vi "Color Pattern Matching.vi"() -> ()   [LabVIEW 2014]
doc: "This example shows how to use the color pattern matching tools in NI Vision.\n\nYou use color pattern matching to locate known reference or fiducial patterns in an image quickly. Pattern matching is the key to many applications. Color pattern matching can provide your application with information about the presence or absence, number, and location of the model within an image.\n\nYou use color pattern matching in the following three general applications areas:\n\n* Alignment -- Determine the position and orientation of a known object by locating features. You use the features as points of reference on the object.\n\n* Gauging -- Measure lengths, diameters, angles, and other critical dimensions. If the measurements fall outside of set tolerance levels, the component is rejected. You sometimes use gauging in-line with the manufacturing process and off-line. If you make the measurements off-line, a sample of components is used to determine the quality of a lot or batch of manufactured components.\n\n* Inspection -- Detect simple flaws, such as missing parts or unreadable printing."
uses:
  <vilib>/vision/NI_Vision_Development_Module.lvlib
panel:
  out "Number of Matches":i32
  out "Results":T1(array[cluster]) {"Position"."Y" format="%.2f"; "Position"."X" format="%.2f"}
  in  "Max # of Matches":i32=5
  in  "Minimum Score":sgl=700.0
  out "Template":T2(plugin-control)
  in  "Stop":bool
  out "Image":T2(plugin-control)
  # "Overview: Demonstrates how to perform Color Pattern Matching using two steps that include learning the color pattern template defined by a Region of Interest (ROI) and then matching the learned template in the image.\nRequirements: Vision Development Software.\nInstructions:\n1. Run the VI.\n2. Draw a ROI in the image to define the template. The learned template is displayed in the Template display and the match results are overlaid on the Image display."
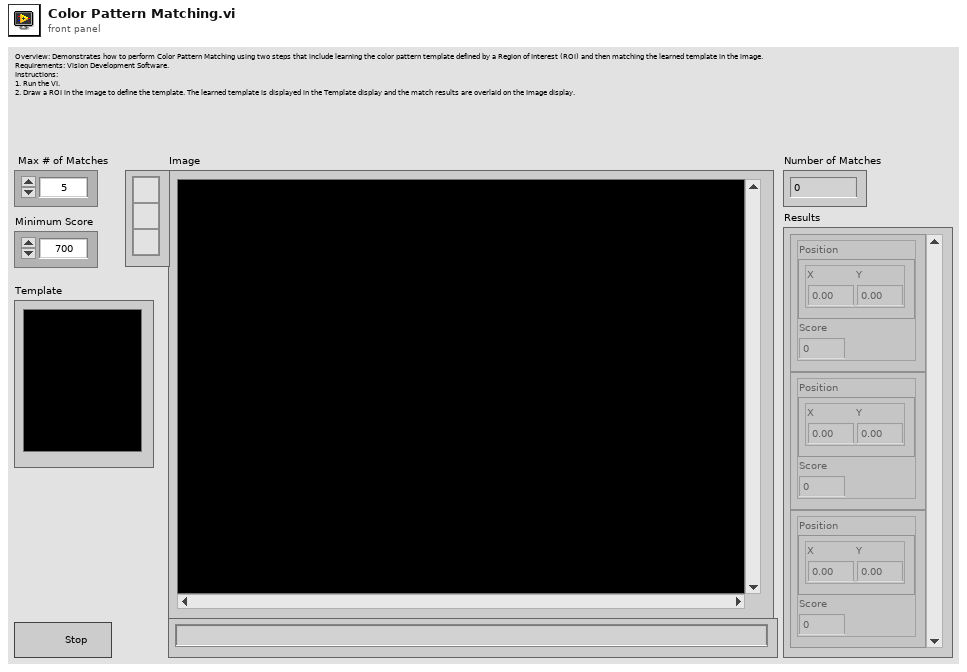
[diagram p1: front panel]
types:
  T1 = cluster{"Position":cluster{"X":dbl, "Y":dbl}, "Score":dbl}[]
  T2 = typedef "IMAQ Image.ctl" = refnum<image>
  T3 = typedef "Image Type" = u32
  T4 = typedef "IMAQ Rectangle" = cluster{"Left":i32, "Top":i32, "Right":i32, "Bottom":i32, "Rotation":dbl}
  T5 = typedef "ROI Descriptor" = cluster{"Global Rectangle":i32[], "Contours":cluster{"ID":enum32{"External", "Internal"}, "Type":u32, "Coordinates":i32[]}[]}
  T6 = cluster{"Max # of Matches":i32, "Minimum Score":sgl}
  T7 = cluster{"Position":cluster{"x":sgl, "y":sgl}, "Angle":sgl, "Scale":sgl, "Score":sgl, "Bounding Box":cluster{"x":sgl, "y":sgl}[]}[]
  T8 = cluster{"Position":cluster{"x":sgl, "y":sgl}, "Score":sgl}
  T9 = cluster{i32[], cluster{"Contour Type":u32, "ROI Type":u32, i32[]}[]}
  T10 = cluster{"Global Rectangle":i32[], "Contours":cluster{"Contour Type":u32, "ROI Type":u32, "Points":i32[]}[]}
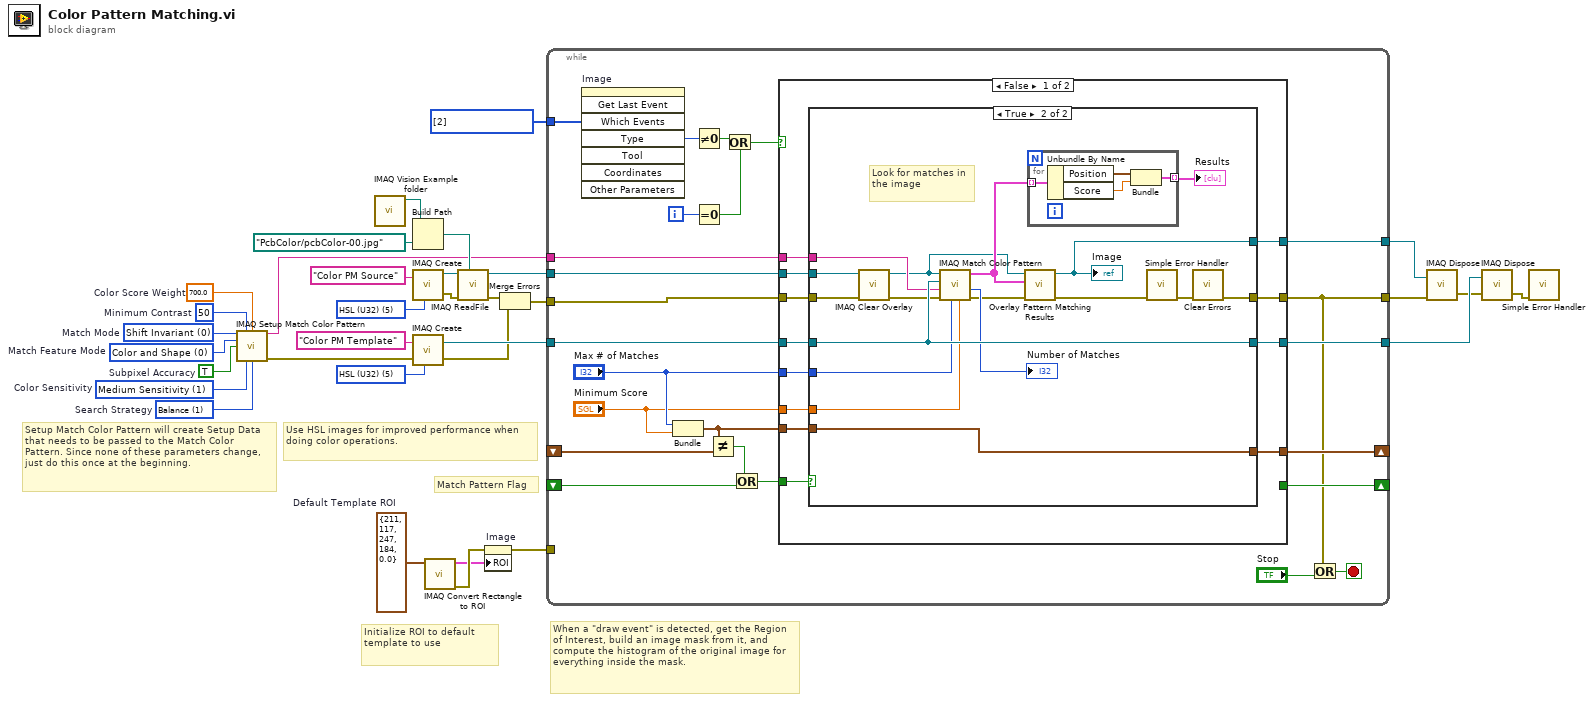
[diagram p0: block diagram]
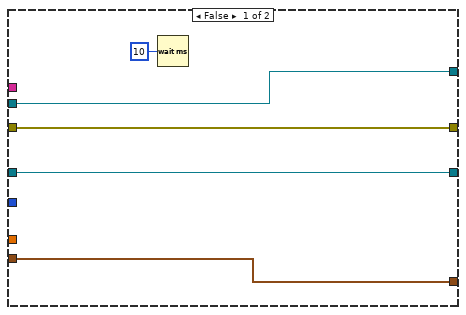
[diagram p2: hidden frame]
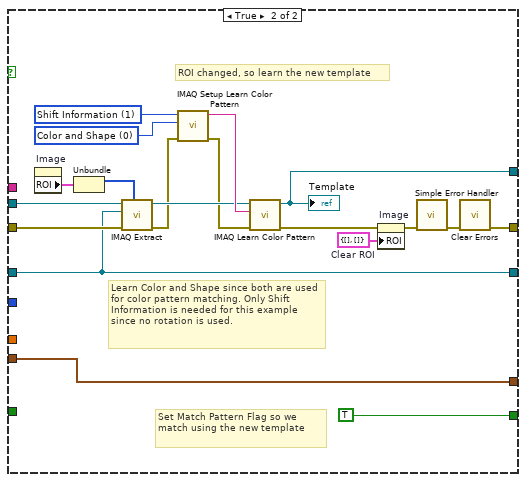
[diagram p3: hidden frame]
diagram:
  w1 = TRUE  # Subpixel Accuracy
  w9 = u32 0 items=["Color and Shape", "Color", "Shape"]  # Match Feature Mode
  w8 = u32 1 items=["Conservative", "Balance", "Aggressive", "Very Aggressive"]  # Search Strategy
  w7 = 50  # Minimum Contrast
  w6 = sgl 700.0  # Color Score Weight
  w5 = u32 1 items=["Low Sensitivity", "Medium Sensitivity", "High Sensitivity"]  # Color Sensitivity
  w4 = u32 0 items=["Shift Invariant", "Rotation Invariant"]  # Match Mode
  w21 = T3 5 items=["Grayscale (U8)", "Grayscale (I16)", "Grayscale (SGL)", "Complex (CSG)", "RGB (U32)", "HSL (U32)", "RGB (U64)", "Grayscale (U16)"] ("Image Type")
  w22 = T3 5 items=["Grayscale (U8)", "Grayscale (I16)", "Grayscale (SGL)", "Complex (CSG)", "RGB (U32)", "HSL (U32)", "RGB (U64)", "Grayscale (U16)"] ("Image Type")
  w27 = i32[] [2] items=["No Event"=0, "Click Event"=1, "Draw Event"=2, "Size Event"=4, "Scroll Event"=5, "Double Click Event"=8] ("Which Events")
  w29 = T4 {"Left"=211, "Top"=117, "Right"=247, "Bottom"=184, "Rotation"=0.0}  # Default Template ROI
  # "Setup Match Color Pattern will create Setup Data that needs to be passed to the Match Color Pattern. Since none of these parameters change, just do this once at the beginning."
  # "Initialize ROI to default template to use"
  # "When a \"draw event\" is detected, get the Region of Interest, build an image mask from it, and compute the histogram of the original image for everything inside the mask."
  # "Match Pattern Flag"
  # "Use HSL images for improved performance when doing color operations."
  n1 = call "IMAQ Setup Match Color Pattern"("Match Mode"=w4, "Minimum Contrast"=w7, "Color Score Weight"=w6, "Match Feature Mode"=w9, "Subpixel Accuracy"=w1, "Color Sensitivity"=w5, "Search Strategy"=w8) -> ("Match Color Pattern Setup Data"=w2:string, "error out"=w3:errorcluster)  [unwired: 7 in]
  n2 = call "IMAQ Vision Example folder.vi"() -> ("Example Image Path"=w32:path)  [unwired: 11 in]
  n3 = Build Path(base path=w32, name or relative path=path "PcbColor/pcbColor-00.jpg") -> (appended path=w28:path)
  n4 = call "IMAQ Create"("Image Name"="Color PM Source", "Image Type"=w22) -> ("New Image"=w13:T2, "error out"=w18:errorcluster)  [unwired: 3 in]
  n5 = call "IMAQ Create"("Image Name"="Color PM Template", "Image Type"=w21, "error in (no error)"=w3) -> ("New Image"=w26:T2, "error out"=w15:errorcluster)  [unwired: 2 in]
  n6 = call "IMAQ Convert Rectangle to ROI"("Rectangle"=w29) -> ("error out"=w17:errorcluster, "ROI Descriptor"=w11:T5)  [unwired: 8 in]
  n7 = call "IMAQ ReadFile"("File Path"=w28, "error in (no error)"=w18, "Image"=w13) -> ("error out"=w16:errorcluster, "Image Out"=w12:T2)  [unwired: 4 in, 3 out]
  n8 = property on="Image" class="ImageControl"(error in=w17, "ROI"=w11) -> (error out=w10:errorcluster)  [unwired: 1 in, 1 out]
  n9 = Merge Errors(w16, w15) -> (w14:errorcluster)
  n10 = while {
    tunnel: w12 -> [w47]
    tunnel: w27 -> [w57]
    tunnel: w26 -> [w46]
    tunnel: w14 -> [w51]
    shift-right: [w45] -> _
    shift-left: _ -> [w38]
    shift-right: [w50] -> _
    shift-left: _ -> [w49]
    tunnel: [w43] -> w25
    tunnel: [w44] -> w24
    tunnel: [w36] -> w23
    tunnel: w10 -> [_]
    tunnel: w2 -> [w40]
    i -> [w54]
    stop <- w34 stop-if-true
    n11 = invoke on="Image" class="ImageControl" method="Get Last Event"("Which Events"=w57) -> ("Type"=w56:i32)  [unwired: 7 in, 7 out]
    n12 = Bundle("Max # of Matches"="Max # of Matches", "Minimum Score"="Minimum Score") -> (w39:T6)  [unwired: 1 in]
    n13 = Not Equal To 0?(x=w56) -> (x != 0?=w55:bool)
    n14 = Equal To 0?(x=w54) -> (x = 0?=w53:bool)
    n15 = Not Equal?(x=w39, y=w38) -> (x != y?=w37:bool)
    n16 = Or(x=w55, y=w53) -> (x .or. y?=w52:bool)
    n17 = Or(x=w37, y=w49) -> (x .or. y?=w48:bool)
    n18 = case shown="False" w52 {
      tunnel: w47 -> [w67 w105]
      tunnel: w51 -> [w66 w104]
      tunnel: w46 -> [w65 w97]
      tunnel: [_ TRUE] -> w50
      tunnel: w48 -> [w69 _]
      tunnel: w39 -> [w68 w96]
      tunnel: [w64 w100] -> w36
      tunnel: [w63 w96] -> w45
      tunnel: [w62 w97] -> w44
      tunnel: [w61 w98] -> w43
      tunnel: "Max # of Matches" -> [w60 _]
      tunnel: "Minimum Score" -> [w59 _]
      tunnel: w40 -> [w58 _]
      frame False {
        n19 = case shown="True" w69 {
          tunnel: w68 -> [w72 w88]
          tunnel: w67 -> [w70 w91]
          tunnel: w66 -> [w74 w90]
          tunnel: w65 -> [w71 w89]
          tunnel: [w74 w86] -> w64
          tunnel: [w72 w88] -> w63
          tunnel: [w71 w89] -> w62
          tunnel: [w70 w76] -> w61
          tunnel: w60 -> [_ w84]
          tunnel: w59 -> [_ w83]
          tunnel: w58 -> [_ w82]
          frame False {
            n20 = Wait (ms)(milliseconds to wait=u32 10) -> ()  [unwired: 1 out]
          }
          frame True {
            # "Look for matches in the image"
            n21 = call "IMAQ Clear Overlay"("error in (no error)"=w90, "Image"=w91) -> ("error out"=w85:errorcluster, "Image Out"=w75:T2)  [unwired: 8 in]
            n22 = call "IMAQ Match Color Pattern"("Minimum Match Score"=w83, "Number of Matches Requested"=w84, "error in (no error)"=w85, "Match Color Pattern Setup Data"=w82, "Template Image"=w89, "Image"=w75) -> ("error out"=w79:errorcluster, "Number of Matches"=→"Number of Matches":i32, "Matches"=w78:T7)  [unwired: 3 in]
            n23 = call "Overlay Pattern Matching Results.vi"("error in"=w79, "Matches"=w78, "Image"=w75) -> ("error out"=w77:errorcluster, "Image Out"=w76:T2)  [unwired: 7 in]
            "Image" <- w76
            n24 = for {
              tunnel: w78 -> [w95] mode=indexing
              tunnel: [w92] -> w81 mode=indexing
              n25 = Unbundle By Name(w95) -> ("Position"=w94:cluster{"x":sgl, "y":sgl}, "Score"=w93:sgl)
              n26 = Bundle("Position"=w94, "Score"=w93) -> (w92:T8)  [unwired: 1 in]
            }
            "Results" <- w81
            n27 = call <vilib>:"Simple Error Handler.vi"("error in (no error)"=w77) -> ("error out"=w87:errorcluster)  [unwired: 4 in, 4 out]
            n28 = call <vilib>:"Clear Errors.vi"("error in (no error)"=w87) -> ("error out"=w86:errorcluster)  [unwired: 5 in, 1 out]
          }
        }
      }
      frame True {
        w102 = u32 0 items=["Color and Shape", "Color", "Shape "] ("Feature Mode")
        w106 = u32 1 items=["All", "Shift Information", "Rotation Information"] ("Learn Mode")
        w107 = T9 {[], []}  # Clear ROI
        # "Set Match Pattern Flag so we match using the new template"
        # "Learn Color and Shape since both are used for color pattern matching. Only Shift Information is needed for this example since no rotation is used."
        # "ROI changed, so learn the new template"
        n29 = property on="Image" class="ImageControl"() -> ("ROI"=w109:T10)  [unwired: 2 in, 2 out]
        n30 = Unbundle(w109) -> ("Global Rectangle"=w114:i32[])  [unwired: 1 out]
        n31 = call "IMAQ Extract"("Optional Rectangle"=w114, "error in (no error)"=w104, "Image Dst"=w97, "Image Src"=w105) -> ("error out"=w111:errorcluster, "Image Dst Out"=w112:T2)  [unwired: 6 in]
        n32 = call "IMAQ Setup Learn Color Pattern"("error in (no error)"=w111, "Feature Mode"=w102, "Learn Mode"=w106) -> ("error out"=w110:errorcluster, "Learn Color Pattern Setup Data"=w113:string)  [unwired: 7 in]
        n33 = call "IMAQ Learn Color Pattern"("error in (no error)"=w110, "Learn Color Pattern Setup Data"=w113, "Image"=w112) -> ("error out"=w99:errorcluster, "Template Image Out"=w98:T2)  [unwired: 7 in]
        "Template" <- w98
        n34 = property on="Image" class="ImageControl"(error in=w99, "ROI"=w107) -> (error out=w108:errorcluster)  [unwired: 1 in, 1 out]
        n35 = call <vilib>:"Simple Error Handler.vi"("error in (no error)"=w108) -> ("error out"=w101:errorcluster)  [unwired: 4 in, 4 out]
        n36 = call <vilib>:"Clear Errors.vi"("error in (no error)"=w101) -> ("error out"=w100:errorcluster)  [unwired: 5 in, 1 out]
      }
    }
    n37 = Or(x=w36, y="Stop") -> (x .or. y?=w34:bool)
  }
  n38 = call "IMAQ Dispose"("Image"=w25, "error in (no error)"=w23) -> ("error out"=w20:errorcluster)  [unwired: 4 in]
  n39 = call "IMAQ Dispose"("Image"=w24, "error in (no error)"=w20) -> ("error out"=w19:errorcluster)  [unwired: 4 in]
  n40 = call <vilib>:"Simple Error Handler.vi"("error in (no error)"=w19) -> ()  [unwired: 4 in, 5 out]
